vi "STA - Wave V4 Host.vi"() -> ()   [LabVIEW 2015]
doc: "The continuous acquisition mode tells the FPGA to acquire points indefinitely until a stop command is issued or until an error is encountered (FIFO overflow, module underflow, and so on). \n\nIn this acquisition mode, explicitly call the appropriate rwfm_ConfigTiming VI and set the host application's data buffer to be many times larger than the read size. The examples use a 10X size by default. If the host application's data buffer fills, then the FPGA experiences a FIFO overflow causing the acquisition to stop."
uses:
  <vilib>/LabVIEW Targets/FPGA/cRIO/shared/nicrio_ModuleControls/nicrio_cRIO-9234_ConfigModeRing.ctl
  <vilib>/FPGAPlugInAG/cRIO-9112/niLvFpga_Open_cRIO-9112.vi
  <vilib>/rvi/interface/common/dynamic/niFpgaDynamicAddResources.vi
  <vilib>/Utility/error.llb/Error Cluster From Error Code.vi
  <vilib>/RVI Host/nirviSupport.llb/nirviErrorClusterFromErrorCode.vi
  <vilib>/rvi/errors/niLvFpgaAdjustHostInterfaceError.vi
  <vilib>/FPGAPlugInAG/Dynamic/niLvFpga_Close_Dynamic.vi
  <vilib>/rvi/interface/nirviOpenFPGA/nirviOpenFPGA.xnode
  FPGA Bitfiles/STA-WaveformV3_FPGATarget2_[FPGA]DeltaSigMa_0miEeT0hA5U.lvbitx
  FPGA/[FPGA] DeltaSig Main V3.vi
  <vilib>/rvi/interface/nirviMethod/nirviMethod.xnode
  <vilib>/rvi/interface/nirviCloseFPGA/nirviCloseFPGA.xnode
  <vilib>/NI/cRIO Wfm/cRIO Wfm.lvlib
  D/Documents/LabVIEW Data/STA - Waveform V0/FPGA Bitfiles/SARAcqMain_9074.lvbitx
  C:/Program Files (x86)/National Instruments/LabVIEW 2015/ProjectTemplates/Source/cRIOWfm/FPGA/[FPGA] SAR Acq Main.vi
  <vilib>/rvi/interface/nirviMethod/StockFPGA_InlinedMethodWaitForSingleIRQ.vi
  <vilib>/FPGAPlugInAG/Dynamic/niLvFpga_WaitOnIrq_Dynamic.vi
panel:
  out "data rate (S/s)":u32
  out "Channel Config":T2(array[cluster]) {"Input Configuration" items=["AC Coupled", "DC Coupled", "IEPE AC Coupled"]}
  out "Samples per Read":i32
  out "file path":path
  in  "error in (no error)":errorcluster
  out "error out":errorcluster
  in  "stop":bool
  out "Waveform Graph":waveform(sgl)[](graph)
  out "Buffer Backlog":dbl caption="RT Buffer Backlog [%]" format="%#.2g"
  # "Sampling Info"
  # "Channel Info"
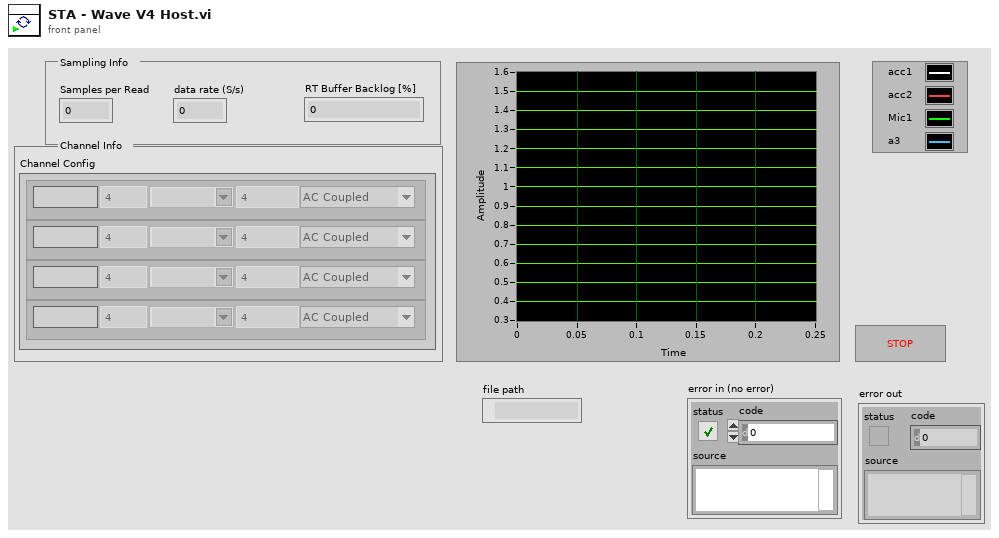
[diagram p1: front panel]
types:
  T1 = typedef "nicrio_cRIO-9234_ConfigModeRing.ctl" = u8
  T2 = cluster{"Channel Name":string, "Sensitivity mV_EU":dbl, "EU":string, "Input Configuration":T1, "dB Ref EU":dbl}[]
  T3 = enum16{"open", "open or create", "create or replace", "create", "open (read-only)"}
  T4 = typedef "Acquisition and Logging Configuration_Waveform.ctl" = cluster{"Data Rate":T5, "Samples per Read":i32, "Number of Reads to Save":i32, "Data File Name":string, "TDMS Properties":T6[], "Number of Channels":i32, "Trigger - RMS Value":dbl, "Trigger - Channel":i32, "Trigger - Time (Minute)":i32, "Channel Config":cluster{"Channel Name":string, "Sensitivity mV_EU":dbl, "EU":string, "Input Configuration":T1, "dB Ref EU":dbl}[], "data rate (S/s)":u32, "Time Measure":dbl}
  T5 = typedef "nicrio_cRIO-9234_DataRatesRing2.ctl" = u8
  T6 = typedef "TDMS Properties.ctl" = cluster{"Name":string, "Value":string}
  T7 = typedef "cRIO Wfm.lvlib/SamplingInfo.ctl" = cluster{"Number of Channels":i32, "Actual Samp Rate":dbl, "Chan Name Array":string[], "EU Chan Array":string[], "dB Ref Chan Array":dbl[]}
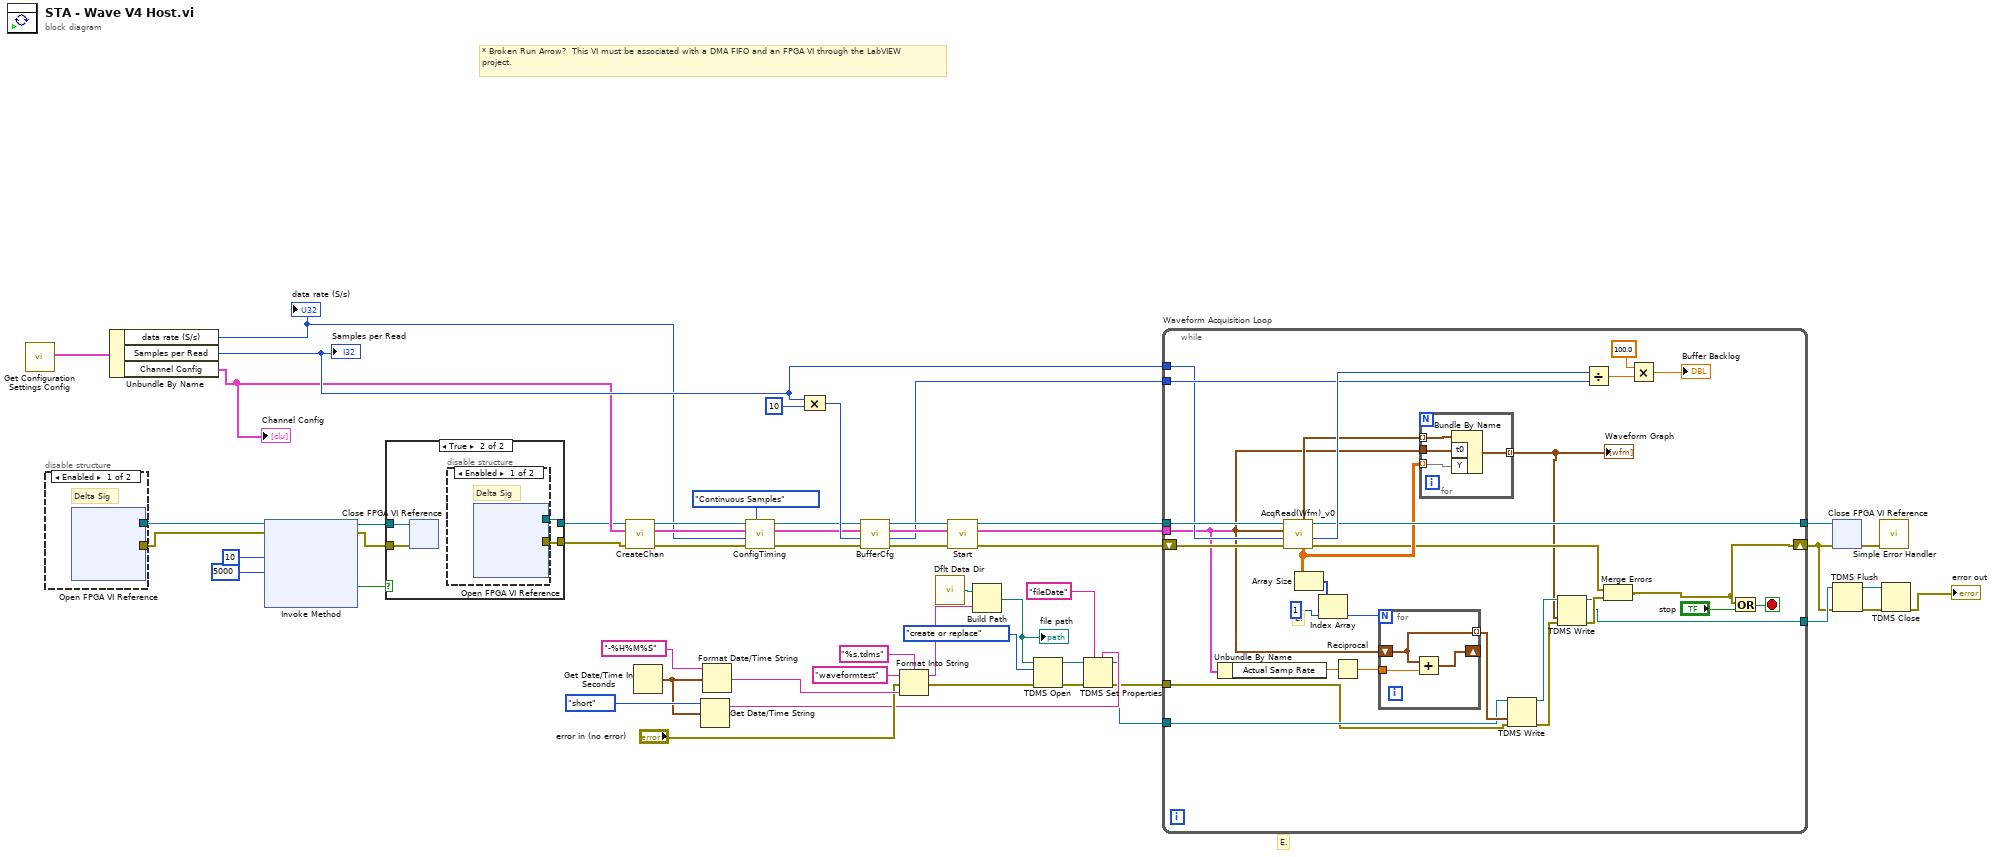
[diagram p0: block diagram]
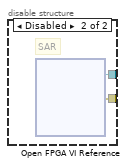
[diagram p3: hidden frame]
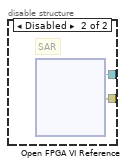
[diagram p4: hidden frame]
diagram:
  # "E."
  # "* Broken Run Arrow?  This VI must be associated with a DMA FIFO and an FPGA VI through the LabVIEW project."
  n1 = call "Get Configuration Settings Config.vi"() -> ("Configuration"=w14:T4)  [unwired: 10 in, 1 out]
  n2 = disable-structure shown="Enabled" {
    disable-tunnel: [w56 w58] -> w8
    disable-tunnel: [w55 w57] -> w7
    frame Enabled {
      # "Delta Sig"
      n3 = xnode "Open FPGA VI Reference"() -> ("FPGA VI Reference Out"=w56:refnum<k20>, "error out"=w55:errorcluster)  [unwired: 2 in]
    }
    frame Disabled {
      # "SAR"
      n4 = xnode "Open FPGA VI Reference"() -> ("FPGA VI Reference Out"=w58:refnum<k20>, "error out"=w57:errorcluster)  [unwired: 2 in]
    }
  }
  n5 = Unbundle By Name(w14) -> ("data rate (S/s)"=w11:u32, "Samples per Read"=w13:i32, "Channel Config"=w12:T2)
  "Samples per Read" <- w13
  "Channel Config" <- w12
  "data rate (S/s)" <- w11
  n6 = xnode "Invoke Method"("FPGA VI Reference In"=w8, "error in"=w7, "IRQ Number(s)"=10, "Timeout (ms)"=5000) -> ("FPGA VI Reference Out"=w5:refnum<k20>, "error out"=w4:errorcluster, "Timed Out"=w6:bool)  [unwired: 1 out]
  n7 = case shown="True" w6 {
    tunnel: w5 -> [w60 w64]
    tunnel: w4 -> [w59 w63]
    tunnel: [w60 w62] -> w3
    tunnel: [w59 w61] -> w2
    frame False {
    }
    frame True {
      n8 = xnode "Close FPGA VI Reference"("FPGA VI Reference In"=w64, "error in"=w63) -> ()  [unwired: 1 out]
      n9 = disable-structure shown="Enabled" {
        disable-tunnel: [w66 w68] -> w62
        disable-tunnel: [w65 w67] -> w61
        frame Enabled {
          # "Delta Sig"
          n10 = xnode "Open FPGA VI Reference"() -> ("FPGA VI Reference Out"=w66:refnum<k20>, "error out"=w65:errorcluster)  [unwired: 2 in]
        }
        frame Disabled {
          # "SAR"
          n11 = xnode "Open FPGA VI Reference"() -> ("FPGA VI Reference Out"=w68:refnum<k20>, "error out"=w67:errorcluster)  [unwired: 2 in]
        }
      }
    }
  }
  n12 = call <vilib>:"CreateChan.vi"("Dynamic FPGA Ref"=w3, "Channel Config"=w12, "error in"=w2) -> ("Dynamic FPGA Ref Out"=w43:refnum<k20>, "Sampling Info"=w42:T7, "error out"=w38:errorcluster)  [unwired: 5 in]
  n13 = Get Date/Time In Seconds() -> (seconds since 1Jan1904=w1:timestamp)
  n14 = Get Date/Time String(date format (0)=enum16{"short", "long", "abbreviated"}."short", seconds (now)=w1) -> (date string=w22:string)  [unwired: 1 in, 1 out]
  n15 = Format Date/Time String(time format string (%c)="-%H%M%S", seconds (now)=w1) -> (date/time string=w32:string)  [unwired: 1 in]
  n16 = call <vilib>:"ConfigTiming.vi"("Sample Mode"=enum16{"Finite Samples", "Continuous Samples"}."Continuous Samples", "error in"=w38, "Sample Rate"=w11, "Sampling Info In"=w42, "Dynamic FPGA Ref"=w43) -> ("error out"=w39:errorcluster, "Sampling Info Out"=w40:T7, "Dynamic FPGA Ref Out"=w41:refnum<k20>)  [unwired: 3 in, 1 out]
  n17 = Compound Arithmetic op=MULTIPLY(w13, 10 ("value")) -> (w47:i32)
  n18 = call <vilib>:"BufferCfg.vi"("error in"=w39, "Buffer Size [Samps per Chan]"=w47, "Sampling Info In"=w40, "Dynamic FPGA Ref"=w41) -> ("error out"=w48:errorcluster, "Buffer Size [Total Samples]"=w44:u32, "Sampling Info Out"=w46:T7, "Dynamic FPGA Ref Out"=w49:refnum<k20>)  [unwired: 4 out]
  n19 = Format Into String(format string="%s.tdms", initial string="waveformtest", error in="error in (no error)", w32) -> (resulting string=w36:string, error out=w20:errorcluster)
  n20 = call <vilib>:"Dflt Data Dir.vi"() -> ("App:Default Data Directory"=w29:path)
  n21 = call <vilib>:"Start.vi"("error in"=w48, "Sampling Info In"=w46, "Dynamic FPGA Ref"=w49) -> ("error out"=w53:errorcluster, "Sampling Info Out"=w45:T7, "Dynamic FPGA Ref Out"=w54:refnum<k20>)  [unwired: 6 out]
  n22 = Build Path(base path=w29, name or relative path=w36) -> (appended path=w25:path)
  "file path" <- w25
  n23 = TDMS Open(8:w20, 10:T3."create or replace" ("operation (0:open)"), 11:w25) -> (0:w28:errorcluster, 3:w27:refnum<k34>)  [unwired: 4 in]
  n24 = TDMS Set Properties(5:w22, 7:"fileDate" ("property names"), 8:w28, 11:w27) -> (0:w18:errorcluster, 3:w19:refnum<k34>)  [unwired: 2 in, 2 out]
  n25 = while "Waveform Acquisition Loop" {
    tunnel: w54 -> [w92]
    tunnel: [w88] -> w52
    tunnel: w45 -> [w84]
    tunnel: w44 -> [w96]
    tunnel: w13 -> [w89]
    shift-right: [w80] -> w16
    shift-left: w53 -> [w98]
    tunnel: w19 -> [w78]
    tunnel: w18 -> [w77]
    tunnel: [w73] -> w17
    stop <- w91 stop-if-true
    # "E."
    n26 = Unbundle By Name(w84) -> ("Actual Samp Rate"=w83:dbl)
    n27 = call <vilib>:"AcqRead(Wfm)_v0.vi"("error in"=w98, "Samps Read per Chan"=w89, "Sampling Info"=w84, "Dynamic FPGA Ref"=w92) -> ("error out"=w81:errorcluster, "Samples Remaining"=w97:u32, "time stamp"=w85:timestamp, "Dynamic FPGA Ref Out"=w88:refnum<k20>, "transposed array"=w86:sgl[][], "Array"=w87:waveform(sgl)[])  [unwired: 2 in]
    n28 = Array Size(array=w86) -> (size(s)=w72:i32[])
    n29 = Index Array(array=w72, index=1) -> (element=w70:i32)
    n30 = Reciprocal(x=w83) -> (1/x=w82:dbl)
    n31 = for {
      N: w70 -> [_]
      shift-right: [w101] -> _
      shift-left: w85 -> [w100]
      tunnel: [w100] -> w79 mode=indexing
      tunnel: w82 -> [w99]
      n32 = Add(x=w100, y=w99) -> (x+y=w101:timestamp)
    }
    n33 = for {
      tunnel: w87 -> [w105] mode=indexing
      tunnel: w85 -> [w104]
      tunnel: [w103] -> w69 mode=indexing
      tunnel: w86 -> [w102] mode=indexing
      n34 = Bundle By Name(cluster=w105, "t0"=w104, "Y"=w102) -> (w103:waveform(sgl))
    }
    "Waveform Graph" <- w69
    n35 = TDMS Write(0:w78, 9:w79, 11:w77) -> (4:w75:refnum<k34>, 15:w76:errorcluster)  [unwired: 3 in, 2 out]
    n36 = TDMS Write(0:w75, 9:w69, 11:w76) -> (4:w73:refnum<k34>, 15:w74:errorcluster)  [unwired: 3 in, 2 out]
    n37 = Divide(x=w97, y=w96) -> (x/y=w95:dbl)
    n38 = Merge Errors(w81, w74) -> (w80:errorcluster)
    n39 = Multiply(x=100.0, y=w95) -> (x*y=→"Buffer Backlog":dbl)
    n40 = Or(x=w80, y="stop") -> (x .or. y?=w91:bool)
  }
  n41 = xnode "Close FPGA VI Reference"("FPGA VI Reference In"=w52, "error in"=w16) -> ("error out"=w50:errorcluster)
  n42 = TDMS Flush(4:w16, 7:w17) -> (0:w26:errorcluster, 3:w15:refnum<k34>)
  n43 = call <vilib>:"Simple Error Handler.vi"("error in (no error)"=w50) -> ()  [unwired: 1 in, 8 out]
  n44 = TDMS Close(8:w26, 11:w15) -> (0:→"error out":errorcluster)  [unwired: 1 out]
